vi "Test_RequestSynchronousData_DoubleXDoubleY_XPublished_XValueReceived.vi"(8 "error in (no error)":errorcluster, 11 "TestCase in":refnum<class "TestRequestSynchronousData.lvclass">) -> (0 "error out":errorcluster, 3 "TestCase out":refnum<class "TestRequestSynchronousData.lvclass">)   [LabVIEW 2020, in "TestRequestSynchronousData.lvclass"]
uses:
  TestRequestSynchronousData.lvclass
  TestRequestSynchronousData.lvclass/TestRequestSynchronousData.ctl
  24bf8875-c008-4f22-9bfa-88e42476d167.vi
  Source/IModel/IModel/IModel.lvclass
  Doubles/RootModelPublishesDoubleFloatX/RootModelPublishesDoubleFloatX.lvclass
  <vilib>/ActorFramework/Actor/Actor.lvclass
  Source/Mediator/Mediator/Mediator.lvclass
  <vilib>/ActorFramework/Stop Msg/Stop Msg.lvclass
  modules/composed-event-logger/Source/String Control Sink/String Control Sink.lvclass
  f7bee35d-b044-4098-91af-55574313c386.vi
  modules/composed-event-logger/Source/Composed Log/LoggerReference/LoggerReference.lvclass
  11850773-0e08-463b-84b0-7f64b956e994.vi
  Doubles/ModelSynchronouslyRequestsDoubleFloat/ModelSynchronouslyRequestsDoubleFloat.lvclass
  C:/Git/mva-core/Source/RootModel/RootModel/RootModel.lvclass
  C:/Git/mva-core/Source/IModel/IModel/IModel.lvclass
  C:/Git/mva-core/Source/IObserver/IObserver/IObserver.lvclass
  C:/Program Files (x86)/National Instruments/LabVIEW 2020/vi.lib/ActorFramework/Actor/Actor.lvclass
  C:/Git/mva-core/Test/Doubles/RootModelPublishesDoubleFloatX/RootModelPublishesDoubleFloatX.lvclass
  C:/Git/mva-core/Test/Doubles/ModelSynchronouslyRequestsDoubleFloat/ModelSynchronouslyRequestsDoubleFloat.lvclass
panel:
  out "Y Request Result":T1
  out "X Request Result":T1
  out "Log":string
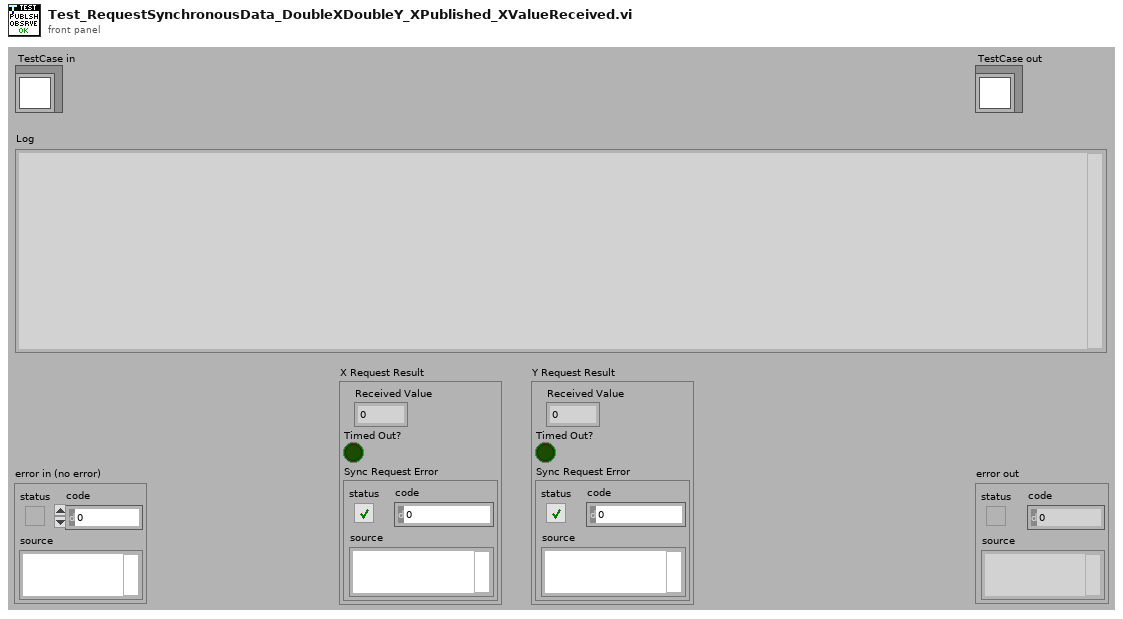
[diagram p1: front panel]
types:
  T1 = cluster{"Received Value":dbl, "Timed Out?":bool, "Sync Request Error":errorcluster}
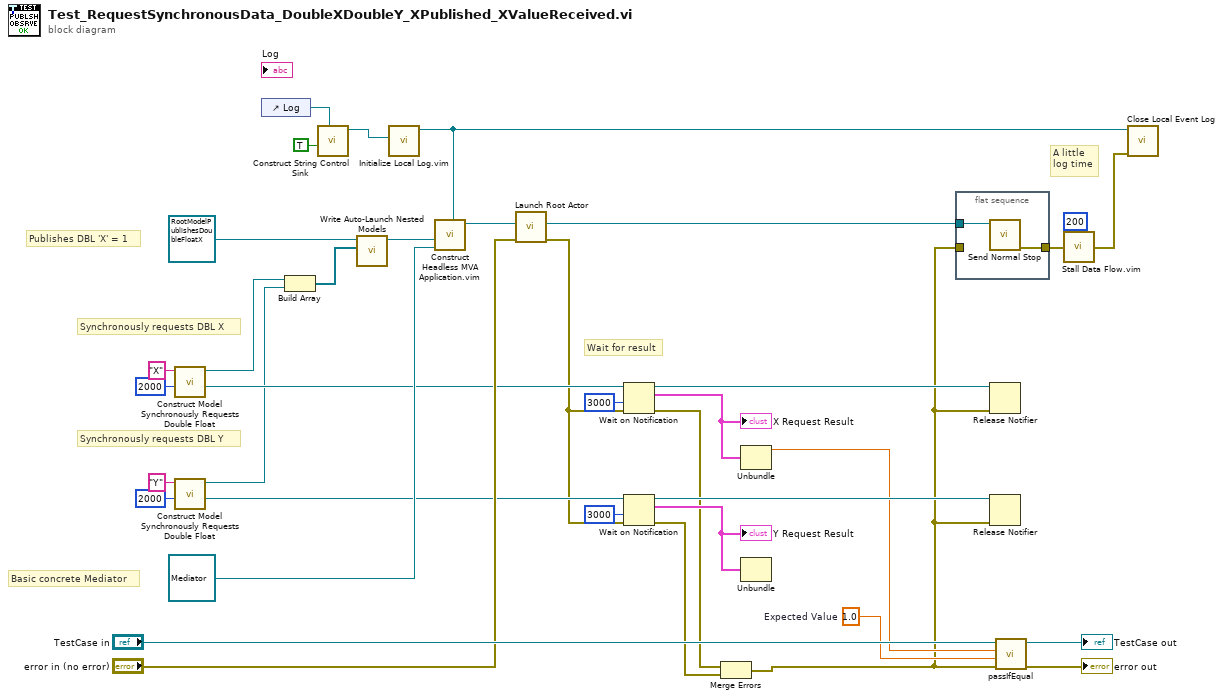
[diagram p0: block diagram]
diagram:
  w26 = 1.0  # Expected Value
  # "Synchronously requests DBL Y"
  # "A little\nlog time"
  # "Wait for result"
  # "Basic concrete Mediator"
  # "Synchronously requests DBL X"
  # "Publishes DBL 'X' = 1"
  n1 = call "Construct Model Synchronously Requests Double Float.vi"("DBL Request Timeout (2000)"=2000, "DBL Name"="X") -> ("Result Notifier"=w23:refnum<notifier>, "ModelSynchronouslyRequestsDoubleFloat Out"=w15:refnum<class "ModelSynchronouslyRequestsDoubleFloat.lvclass">)  [unwired: 8 in]
  n2 = call "Construct Model Synchronously Requests Double Float.vi"("DBL Request Timeout (2000)"=2000, "DBL Name"="Y") -> ("Result Notifier"=w6:refnum<notifier>, "ModelSynchronouslyRequestsDoubleFloat Out"=w2:refnum<class "ModelSynchronouslyRequestsDoubleFloat.lvclass">)  [unwired: 8 in]
  n3 = control-ref of="Log"() -> (w22:refnum<vi>)
  n4 = Build Array(w15, w2) -> (w32:refnum<class "ModelSynchronouslyRequestsDoubleFloat.lvclass">[])
  n5 = call "Construct String Control Sink.vi"("Str Refnum"=w22, "AutoScroll?(F)"=TRUE) -> ("String Control Sink out"=w21:refnum<class "String Control Sink.lvclass">)  [unwired: 9 in]
  n6 = call "Write Auto-Launch Nested Models.vi"("Auto-Launch Nested Models"=w32, "IModel In"=refnum<class "RootModelPublishesDoubleFloatX.lvclass"> refnum ("RootModelPublishesDoubleFloatX.lvclass")) -> ("IModel Out"=w31:refnum<class "RootModelPublishesDoubleFloatX.lvclass">)  [unwired: 9 in]
  n7 = call "Initialize Local Log.vim"("Startup Sink(s)"=w21) -> ("Log Instance Reference"=w19:refnum<class "LoggerReference.lvclass">)  [unwired: 8 in, 2 out]
  n8 = call "Construct Headless MVA Application.vim"("Parent Log Reference"=w19, "Mediator Type"=refnum<class "Mediator.lvclass"> refnum ("Mediator.lvlib:Mediator.lvclass"), "RootModel in"=w31) -> ("RootModel out"=w30:refnum<class "RootModelPublishesDoubleFloatX.lvclass">)  [unwired: 8 in]
  n9 = call <vilib>:"Launch Root Actor.vi"("error in (no error)"="error in (no error)", "Actor"=w30) -> ("error out"=w5:errorcluster, "Actor's Enqueuer"=w25:refnum<class "Message Enqueuer.lvclass">)  [unwired: 8 in]
  n10 = Wait on Notification(notifier=w23, timeout in ms (-1)=3000, error in (no error)=w5) -> (notifier out=w29:refnum<notifier>, notification=w11:T1, error out=w4:errorcluster)  [unwired: 1 in, 1 out]
  "X Request Result" <- w11
  n11 = Wait on Notification(notifier=w6, timeout in ms (-1)=3000, error in (no error)=w5) -> (notifier out=w37:refnum<notifier>, notification=w8:T1, error out=w3:errorcluster)  [unwired: 1 in, 1 out]
  "Y Request Result" <- w8
  n12 = Merge Errors(w4, w3) -> (w1:errorcluster)
  n13 = Unbundle(w11) -> ("Received Value"=w12:dbl)  [unwired: 2 out]
  n14 = Unbundle(w8) -> ()  [unwired: 3 out]
  n15 = flat-sequence {
    tunnel: w25 -> [w39]
    tunnel: [w38] -> w18
    tunnel: w1 -> [_]
    frame #0 {
      n16 = call <vilib>:"Send Normal Stop.vi"("Message Enqueuer"=w39) -> ("error out"=w38:errorcluster)  [unwired: 10 in]
    }
  }
  n17 = Release Notifier(notifier=w29, error in (no error)=w1) -> ()  [unwired: 1 in, 3 out]
  n18 = Release Notifier(notifier=w37, error in (no error)=w1) -> ()  [unwired: 1 in, 3 out]
  n19 = call-dynamic "passIfEqual.vi"("error in (no error)"=w1, "y"=w26, "x"=w12, "TestCase in"="TestCase in") -> ("error out"=→"error out":errorcluster, "TestCase out"=→"TestCase out":refnum<class "TestRequestSynchronousData.lvclass">)  [unwired: 6 in]
  n20 = call "Stall Data Flow.vim"("value in"=w18, "milliseconds to wait"=u32 200) -> ("value out"=w17:errorcluster)  [unwired: 1 out]
  n21 = call "Close Local Event Log.vi"("error in (no error)"=w17, "Log Instance"=w19) -> ()  [unwired: 9 in, 1 out]
